vi "pochodna- test.vi"() -> ()   [LabVIEW 2013]
uses:
  <vilib>/measure/NI_MABase.lvlib
  <vilib>/Analysis/NI_AALPro.lvlib
panel:
  in  "Active Y Scale":i32
  out "Waveform Graph 2":dbl[](graph)
  out "Funkcja Graph":waveform(dbl)[](graph)
  in  "signal type":T1(ring)
  out "Waveform Graph":waveform(dbl)[](graph)
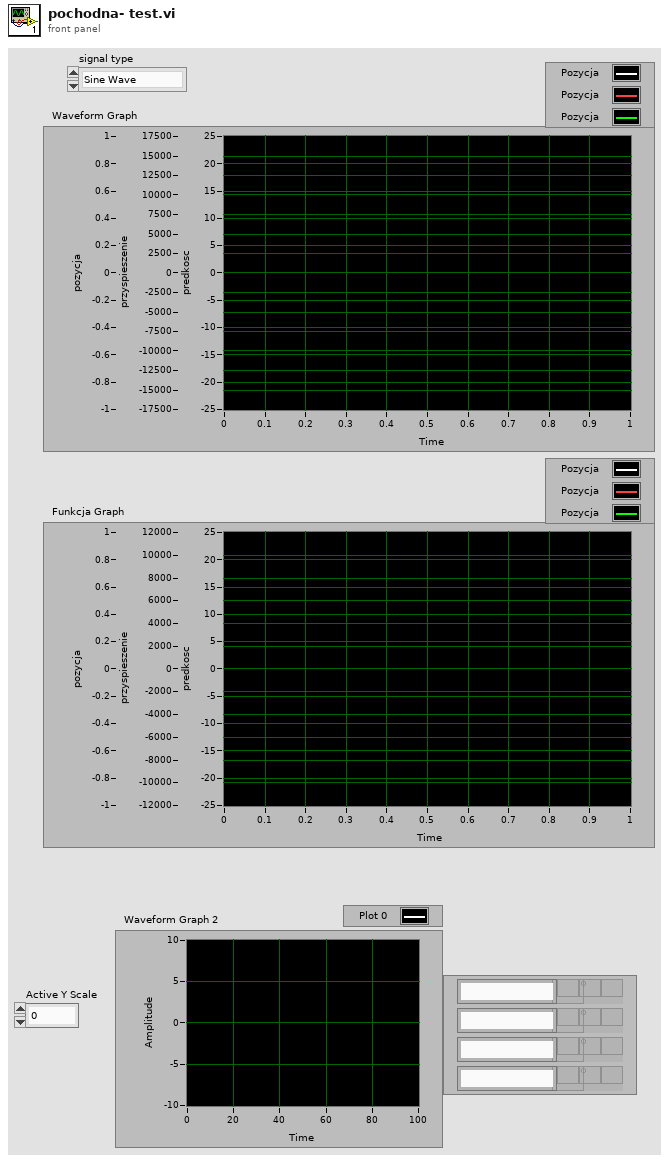
[diagram p1: front panel]
types:
  T1 = enum16{"Sine Wave", "Triangle Wave", "Square Wave", "Sawtooth Wave"}
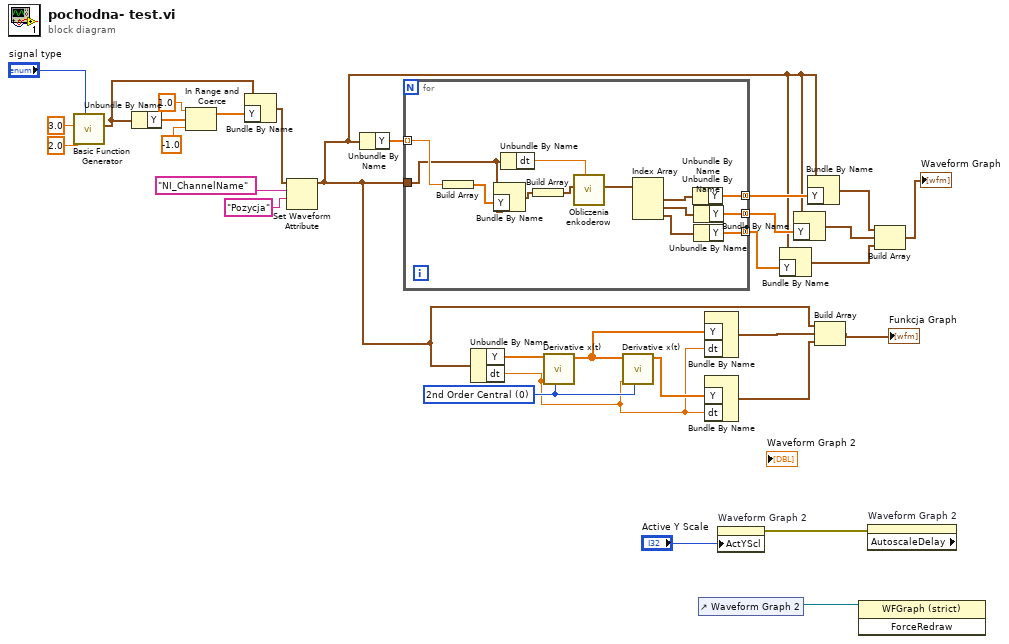
[diagram p0: block diagram]
diagram:
  w17 = u16 0 items=["2nd Order Central", "4th Order Central", "Forward", "Backward"] ("method")
  n1 = call <vilib>:"Basic Function Generator.vi"("signal type"="signal type", "amplitude"=3.0, "frequency"=2.0) -> ("signal out"=w7:waveform(dbl))  [unwired: 6 in, 2 out]
  n2 = Unbundle By Name(w7) -> ("Y"=w10:dbl[])
  n3 = In Range and Coerce(upper limit=1.0, x=w10, lower limit=-1.0) -> (coerced(x)=w9:dbl[])  [unwired: 1 out]
  n4 = Bundle By Name(cluster=w7, "Y"=w9) -> (w8:waveform(dbl))
  n5 = Set Waveform Attribute(5:"Pozycja" ("name"), 6:"NI_ChannelName" ("name"), 7:w8) -> (3:w16:waveform(dbl))  [unwired: 1 in, 2 out]
  n6 = Unbundle By Name(w16) -> ("Y"=w28:dbl[])
  n7 = for {
    tunnel: w28 -> [w44] mode=indexing
    tunnel: w16 -> [w42]
    tunnel: [w34] -> w27 mode=concatenating
    tunnel: [w33] -> w25 mode=concatenating
    tunnel: [w32] -> w26 mode=concatenating
    n8 = Build Array(w44) -> (w41:dbl[])
    n9 = Bundle By Name(cluster=w42, "Y"=w41) -> (w40:waveform(dbl))
    n10 = Unbundle By Name(w42) -> ("dt"=w43:dbl)
    n11 = Build Array(w40) -> (w39:waveform(dbl)[])
    n12 = call "Obliczenia enkoderow.vi"("dT"=w43, "Enkoder in"=w39) -> ("Enkoder out"=w38:waveform(dbl)[])  [unwired: 8 in, 1 out]
    n13 = Index Array(array=w38) -> (element #1=w37:waveform(dbl), element #2=w36:waveform(dbl), element #3=w35:waveform(dbl))  [unwired: 3 in]
    n14 = Unbundle By Name(w37) -> ("Y"=w34:dbl[])
    n15 = Unbundle By Name(w36) -> ("Y"=w33:dbl[])
    n16 = Unbundle By Name(w35) -> ("Y"=w32:dbl[])
  }
  n17 = Unbundle By Name(w16) -> ("Y"=w20:dbl[], "dt"=w12:dbl)
  n18 = call <vilib>:"Derivative x(t).vi"("method"=w17, "dt"=w12, "X"=w20) -> ("dX/dt"=w19:dbl[])  [unwired: 7 in, 1 out]
  n19 = call <vilib>:"Derivative x(t).vi"("method"=w17, "dt"=w12, "X"=w19) -> ("dX/dt"=w18:dbl[])  [unwired: 7 in, 1 out]
  n20 = control-ref of="Waveform Graph 2"() -> (w1:refnum<vi>)
  n21 = Bundle By Name("Y"=w19, "dt"=w12) -> (w15:waveform(dbl))  [unwired: 1 in]
  n22 = Bundle By Name("Y"=w18, "dt"=w12) -> (w14:waveform(dbl))  [unwired: 1 in]
  n23 = property on="Waveform Graph 2" class="WFGraph (strict)"("ActYScl"="Active Y Scale") -> (error out=w2:errorcluster)  [unwired: 2 in, 1 out]
  n24 = Bundle By Name(cluster=w16, "Y"=w26) -> (w22:waveform(dbl))
  n25 = Bundle By Name(cluster=w16, "Y"=w25) -> (w23:waveform(dbl))
  n26 = Bundle By Name(cluster=w16, "Y"=w27) -> (w24:waveform(dbl))
  n27 = Build Array(w16, w15, w14) -> (→"Funkcja Graph":waveform(dbl)[])
  n28 = invoke class="WFGraph (strict)" method="ForceRedraw"(reference=w1) -> ()  [unwired: 2 in, 3 out]
  n29 = property on="Waveform Graph 2" class="WFGraph (strict)" props=["AutoscaleDelay"](error in=w2) -> ()  [unwired: 1 in, 3 out]
  n30 = Build Array(w24, w23, w22) -> (→"Waveform Graph":waveform(dbl)[])
